vi "Insert build.vi"(10 "Application":T1={"App Name"="", "Build Type"=enum."Build", "Current Version"="", "Next Version"="", "Check"=FALSE}, 11 "Builder in":refnum<class "Builder.lvclass">) -> (3 "Builder out":refnum<class "Builder.lvclass">)   [LabVIEW 2021, in "App-Builder Library.lvlib" / "Builder.lvclass"]
uses:
  Builder.lvclass
  App descriptions.ctl
  Build Type.ctl
  Builder.lvclass/Builder.ctl
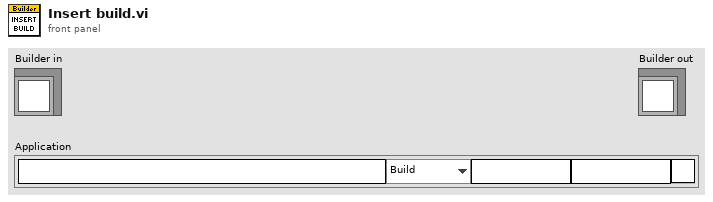
[diagram p1: front panel]
types:
  T1 = typedef "App-Builder Library.lvlib/Builder.lvclass/App descriptions.ctl" = cluster{"App Name":string, "Build Type":T2, "Current Version":string, "Next Version":string, "Check":bool}
  T2 = typedef "App-Builder Library.lvlib/Builder.lvclass/Build Type.ctl" = enum16{"Major", "Minor", "Fix", "Build"}
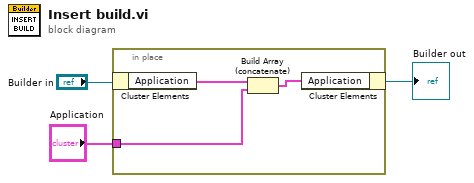
[diagram p0: block diagram]
diagram:
  n1 = in-place {
    in-place-border: "Application" -> [w5]
    n2 = in-place-cluster #1("Builder in") -> ("Application"=w6:T1[])
    n3 = Build Array (concatenate)(w6, w5) -> (w4:T1[])
    n4 = in-place-cluster #1("Application"=w4) -> (→"Builder out":refnum<class "Builder.lvclass">)
  }
